vi "Configuration File Path -- Constant.vi"() -> (2 "Configuration File Path":path)   [LabVIEW 2021]
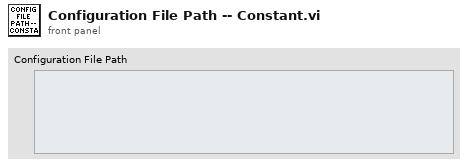
[diagram p1: front panel]
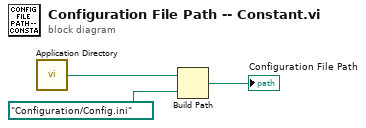
[diagram p0: block diagram]
diagram:
  n1 = call <vilib>:"Application Directory.vi"() -> ("Application Directory"=w3:path)
  n2 = Build Path(base path=w3, name or relative path=path "Configuration/Config.ini") -> (appended path=→"Configuration File Path":path)
